vi "UTILITY Add TC Calibration.vi"(7 "Enum":T1, 10 "TC Coefficients":T2, 11 "Non Cal Temp":dbl) -> (3 "Calibrated Temp":dbl)   [LabVIEW 2016]
uses:
  Type Definitions/UTILITY TC Coefficients.ctl
  Type Definitions/UTILITY TC Coefficients Selector.ctl
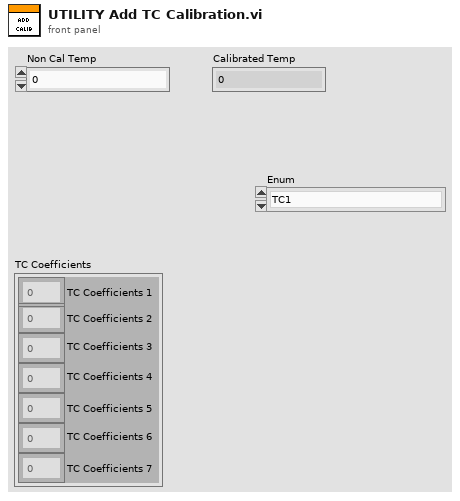
[diagram p1: front panel]
types:
  T1 = typedef "UTILITY TC Coefficients Selector.ctl" = enum16{"TC1", "TC2", "TC3", "TC4", "TC5", "TC6", "TC7"}
  T2 = typedef "UTILITY TC Coefficients.ctl" = cluster{"TC Coefficients 1":dbl[], "TC Coefficients 2":dbl[], "TC Coefficients 3":dbl[], "TC Coefficients 4":dbl[], "TC Coefficients 5":dbl[], "TC Coefficients 6":dbl[], "TC Coefficients 7":dbl[]}
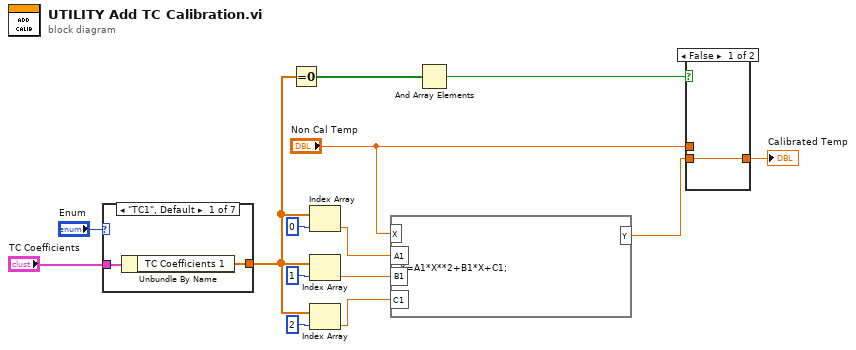
[diagram p0: block diagram]
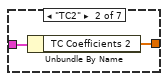
[diagram p3: hidden frame]
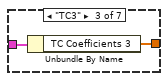
[diagram p4: hidden frame]
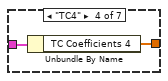
[diagram p5: hidden frame]
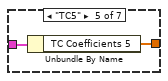
[diagram p6: hidden frame]
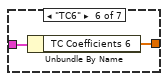
[diagram p7: hidden frame]
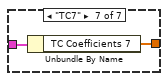
[diagram p8: hidden frame]
diagram:
  n1 = case shown="\"TC1\", Default" "Enum" {
    tunnel: [w16 w17 w19 w21 w23 w25 w27] -> w6
    tunnel: "TC Coefficients" -> [w15 w18 w20 w22 w24 w26 w28]
    frame "TC1", Default {
      n2 = Unbundle By Name(w15) -> ("TC Coefficients 1"=w16:dbl[])
    }
    frame "TC2" {
      n3 = Unbundle By Name(w18) -> ("TC Coefficients 2"=w17:dbl[])
    }
    frame "TC3" {
      n4 = Unbundle By Name(w20) -> ("TC Coefficients 3"=w19:dbl[])
    }
    frame "TC4" {
      n5 = Unbundle By Name(w22) -> ("TC Coefficients 4"=w21:dbl[])
    }
    frame "TC5" {
      n6 = Unbundle By Name(w24) -> ("TC Coefficients 5"=w23:dbl[])
    }
    frame "TC6" {
      n7 = Unbundle By Name(w26) -> ("TC Coefficients 6"=w25:dbl[])
    }
    frame "TC7" {
      n8 = Unbundle By Name(w28) -> ("TC Coefficients 7"=w27:dbl[])
    }
  }
  n9 = Equal To 0?(x=w6) -> (x = 0?=w5:bool[])
  n10 = Index Array(array=w6, index=0) -> (element=w12:dbl)
  n11 = Index Array(array=w6, index=1) -> (element=w13:dbl)
  n12 = Index Array(array=w6, index=2) -> (element=w14:dbl)
  n13 = formula code="Y=A1*X**2+B1*X+C1;"("X"="Non Cal Temp", "A1"=w12, "B1"=w13, "C1"=w14) -> ("Y"=w3:dbl)
  n14 = And Array Elements(Boolean array=w5) -> (logical AND=w4:bool)
  n15 = case shown="False" w4 {
    tunnel: w3 -> [w29 _]
    tunnel: "Non Cal Temp" -> [_ w30]
    tunnel: [w29 w30] -> w1
    frame False {
    }
    frame True {
    }
  }
  "Calibrated Temp" <- w1
